vi "HardwareConfiguration.vi"() -> (3 "configured?":bool=TRUE)   [LabVIEW 2018]
uses:
  InstrControl/InstrumentSetup.vi
  globals/QC_RunInformation.vi
  InstrControl/InstrControl.lvclass
panel:
  in  "RC Configuration":u16(ring) items=["serial", "parallel"]
  in  "AC amplitude [V]":sgl=0.1
  in  "AC frequency [Hz]":i32=1000 format="%#.3p"
  in  "Matrix Configurations":bool
  in  "Defaults Multimeter":bool
  in  "Multimeter":enum32{"Keithley 2000"}(tab)
  in  "Range Value\n(0.1 - 100)":dbl=100.0 format="%#.2g"
  in  "Range":u16(ring) items=["Auto", "Manual"]
  in  "Function":u16(ring)=3 items=["AC Current", "DC Current", "AC Voltage", "DC Voltage", "2W-Resistance", "4W-Resistance", "Period", "Frequency", "Temperature", "Diode", "Continuity"]
  in  "Address KE2000":refnum<visa-resource-name>="GPIB0::19::INSTR"
  in  "Defaults LCR":bool
  in  "LCRs":T1(tab)=enum."HP4284A"
  in  "Address WK6440B":refnum<visa-resource-name>="GPIB0::6::INSTR"
  in  "Address WK6425":refnum<visa-resource-name>
  in  "Address HP4284A":refnum<visa-resource-name>="GPIB0::13::INSTR"
  in  "Consider OC":bool
  in  "Consider SC":bool
  in  "VISA address":refnum<visa-resource-name>="COM4" caption="Arduino address"
  out "Programm uploaded?":string="Make sure programme is uploaded to Arduino Uno ->"
  in  "Blank Button":bool
  in  "Supplies":T2(tab)=enum."Keithley 237"
  in  "Current Limit [µA]":sgl=100.0
  in  "Address KE2410":refnum<visa-resource-name>="GPIB0::16::INSTR"
  in  "Address KE487":refnum<visa-resource-name>
  in  "Compliance":u16(ring) items=["20µA", "2mA"]
  in  "Range:":u16(ring) items=["Autorange", "2nA", "20nA", "200nA", "2 microAmp", "20 microAmp", "200 microAmp", "2 milliAmp"]
  in  "Current Limit":u16(ring)=1 items=["OFF", "ON"]
  in  "Address KE6517":refnum<visa-resource-name>
  in  "current compliance \nlevel [mA]":dbl=0.0001 format="%.4f"
  in  "compliance/measurement\nrange (auto:0)":u16(ring)=6 items=["auto / auto", "1 nA / 1.1 V", "10 nA / 11 V", "100 nA / 110 V", "0.001 mA / 110 V", "0.01 mA / 110 V", "0.1 mA / 110 V", "1 mA / 110 V", "10 mA / 110 V", "100 mA / 110 V"]
  in  "Address KE236":refnum<visa-resource-name>
  in  "Address KE237":refnum<visa-resource-name>="GPIB0::16::INSTR"
  in  "current compliance \nlevel [uA] K237":dbl=10.0 caption="current compliance\nlevel [uA]" format="%.4f"
  in  "compliance/measurement\nrange (auto:0) K237":u16(ring) caption="compliance/measurement\nrange (auto:0)" items=["auto / auto", "1 nA / 1.1 V", "10 nA / 11 V", "100 nA / 110 V", "1 uA / 1100 V", "10 uA / *", "100 uA / *", "1 mA / *", "10 mA / *", "100 mA / *"]
  in  "Defaults Supply":bool
  in  "OK Button":bool
  # "Hardware Configuration"
  # "Multimeter Configuration"
  # "Supply Configuration"
  # "Arduino Configuration"
  # "LCR Configuration"
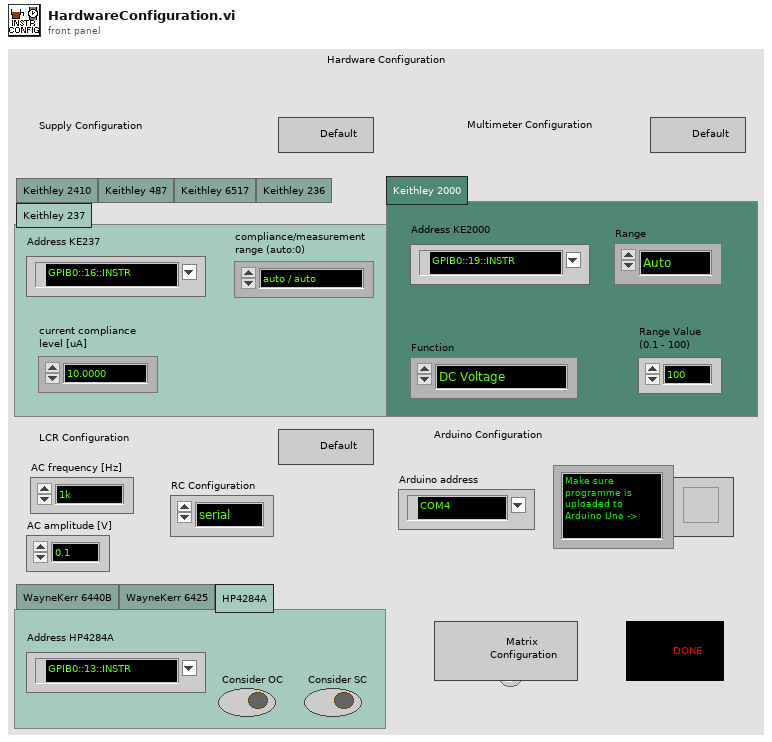
[diagram p1: front panel]
types:
  T1 = enum32{"WayneKerr 6440B", "WayneKerr 6425", "HP4284A"}
  T2 = enum32{"Keithley 2410", "Keithley 487", "Keithley 6517", "Keithley 236", "Keithley 237"}
  T3 = enum16{"CPD", "CPQ", "CPG", "CPRP", "CSD", "CSQ", "CSRS", "LPQ", "LPD", "LPG", "LPRP", "LSD", "LSQ", "LSRS", "RX", "ZTD", "ZTR", "GB", "YTD", "YTR"}
  T4 = cluster{"KE 2410":cluster{"Instrument name":string, "address":refnum<visa-resource-name>, "Instrument type":u16}, "KE 6517":cluster{"Instrument name":string, "address":refnum<visa-resource-name>, "Instrument type":u16}, "KE 487":cluster{"Instrument name":string, "address":refnum<visa-resource-name>, "Instrument type":u16}, "KE 236":cluster{"Instrument name":string, "address":refnum<visa-resource-name>, "Instrument type":u16}, "WK 6440B":cluster{"Instrument name":string, "address":refnum<visa-resource-name>, "Instrument type":u16}, "WK 6425":cluster{"Instrument name":string, "address":refnum<visa-resource-name>, "Instrument type":u16}, "Pickering Matrix":cluster{"Instrument name":string, "address":refnum<visa-resource-name>, "Instrument type":u16}, "KE 2000":cluster{"Instrument name":string, "address":refnum<visa-resource-name>, "Instrument type":u16}, "KE3706A Switching":cluster{"Instrument name":string, "address":refnum<visa-resource-name>, "Instrument type":u16}, "HP 4284A":cluster{"Instrument name":string, "address":refnum<visa-resource-name>, "Instrument type":u16}, "KE237":cluster{"Instrument name":string, "address":refnum<visa-resource-name>, "Instrument type":u16}}
  T5 = cluster{"RC Configuration":u16, "AC amplitude [V]":dbl, "AC frequency [Hz]":i32, "HP 4284A Configurations":cluster{"Consider OC":bool, "Consider SC":bool}}
  T6 = cluster{"VISA address":refnum<visa-resource-name>, "T sensor":enum16{"SHT", "DS"}, "Arduino":refnum<class "ArduinoControl.lvclass">}
  T7 = cluster{"Range":u16, "Range Value":dbl, "Function":u16, "KE2000":refnum<class "KE2000.lvclass">}
  T8 = cluster{"Current Limit":sgl, "KE2410":refnum<class "KE2410.lvclass">}
  T9 = cluster{"Compliance":u16, "Range:":u16, "KE487":refnum<class "KE487.lvclass">}
  T10 = cluster{"Current Limit":u16, "KE6517":refnum<class "KE6517.lvclass">}
  T11 = cluster{"current \ncompliance level":dbl, "compliance/\nmeasurement range (auto:0)":u16, "KE236":refnum<class "KE236.lvclass">}
  T12 = cluster{"current \ncompliance level":dbl, "compliance/\nmeasurement range (auto:0)":u16, "KE237":refnum<class "KE237.lvclass">}
  T13 = cluster{"Sensor Serial No.:":string, "Wafer:":string, "Batch:":string, "Manufacturer:":string, "Device Category:":string, "Database Serial No.:":string, "Date Initiated:":string, "Time Initiated:":string, "Test":string, "Probeplan used:":string, "End of Run Status":dbl, "End of Run comment:":string, "User:":string, "Vbias SMU":string, "LCR":string, "Test SMU":string, "Test DMM":string, "Comments":string, "Measurement results":cluster{"IV":string, "CV":string, "Cis":string, "Ris":string, "Stability":string, "PTP":string, "Striptest":string}}
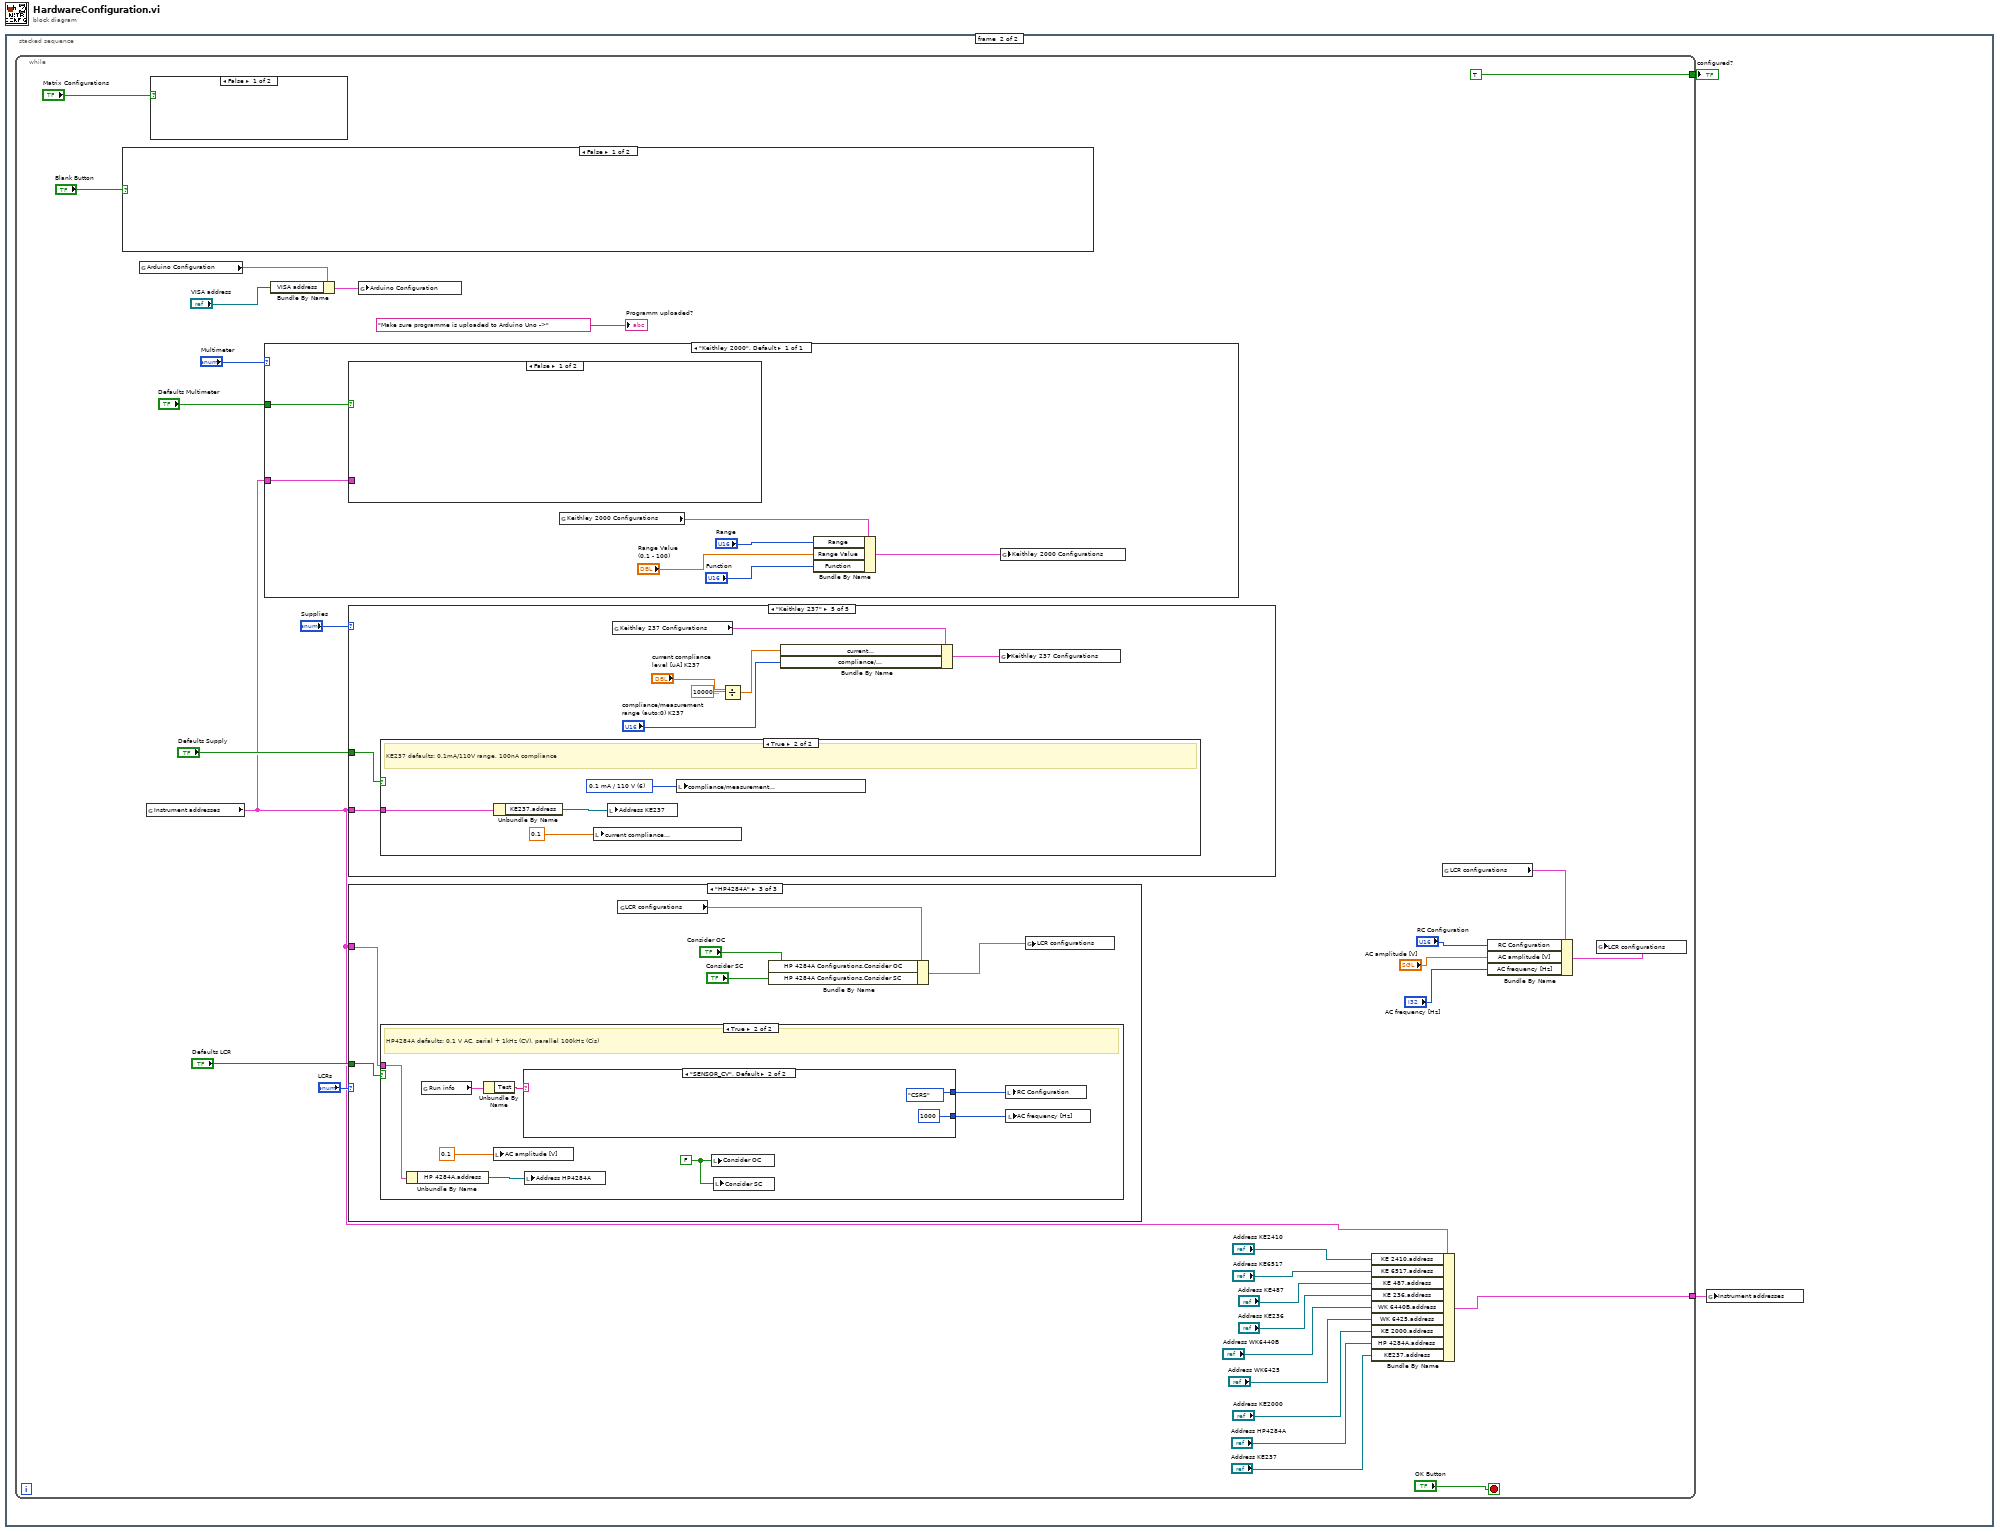
[diagram p0: block diagram]
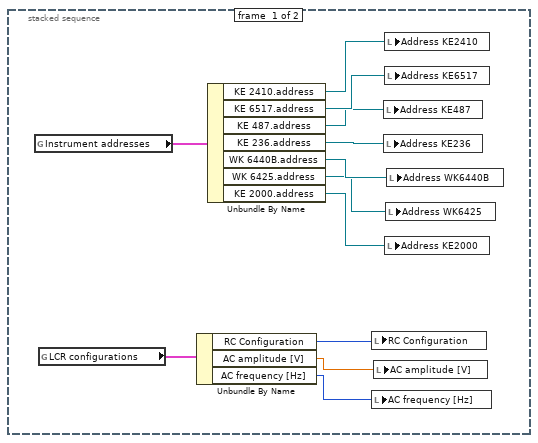
[diagram p2: hidden frame]
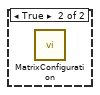
[diagram p3: hidden frame]
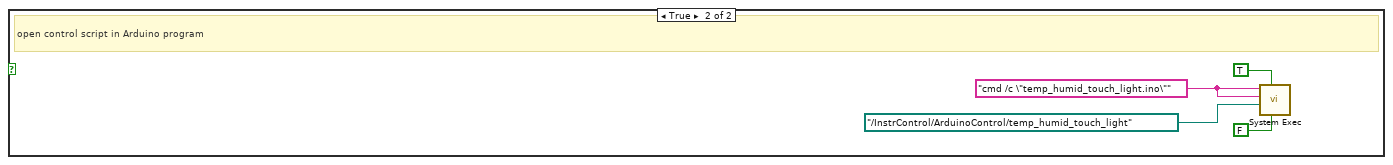
[diagram p4: hidden frame]
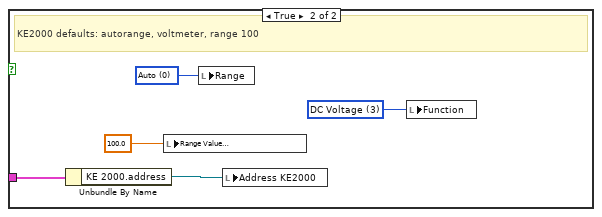
[diagram p5: hidden frame]
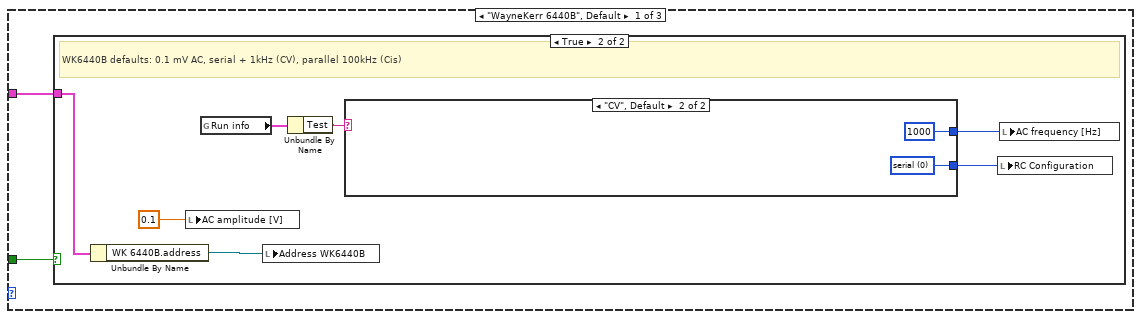
[diagram p6: hidden frame]
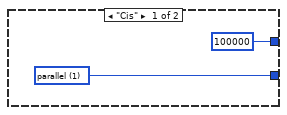
[diagram p8: hidden frame]
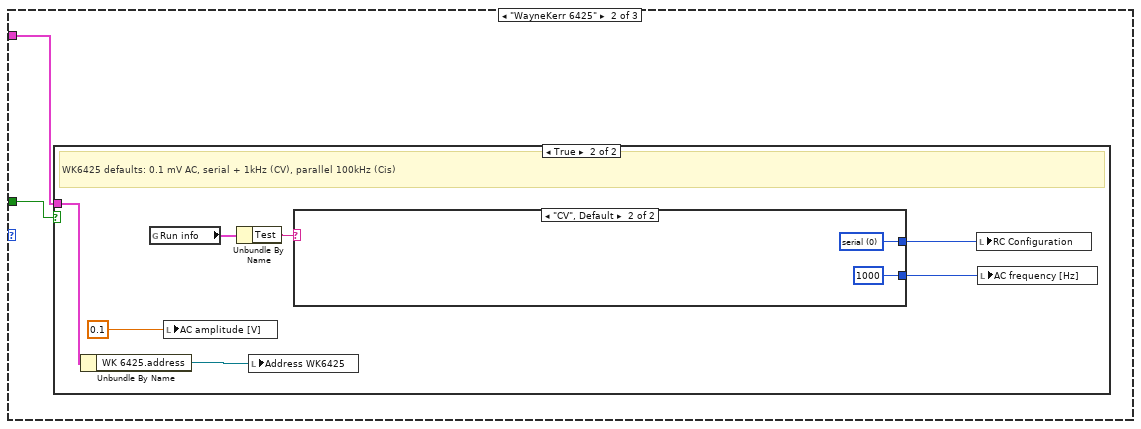
[diagram p9: hidden frame]
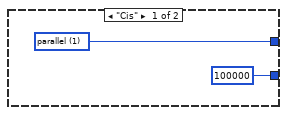
[diagram p11: hidden frame]
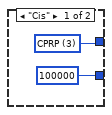
[diagram p13: hidden frame]
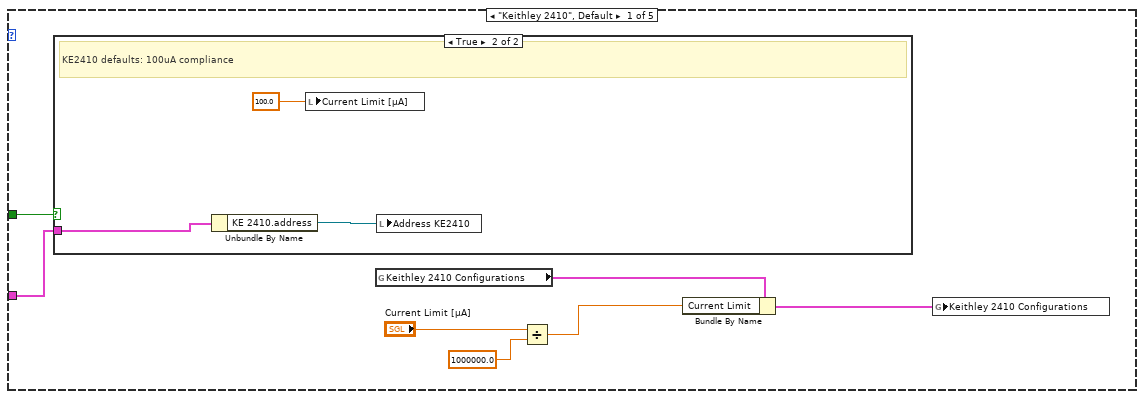
[diagram p14: hidden frame]
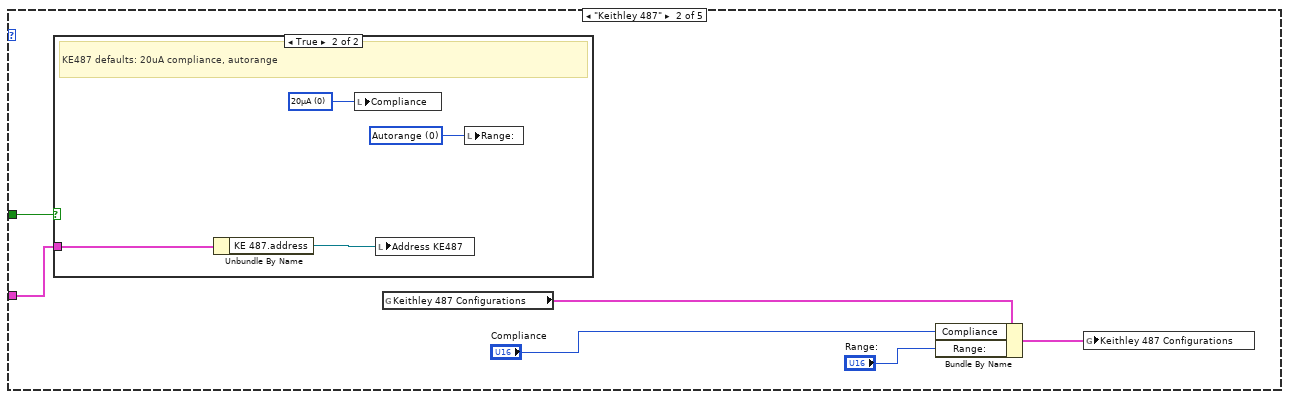
[diagram p16: hidden frame]
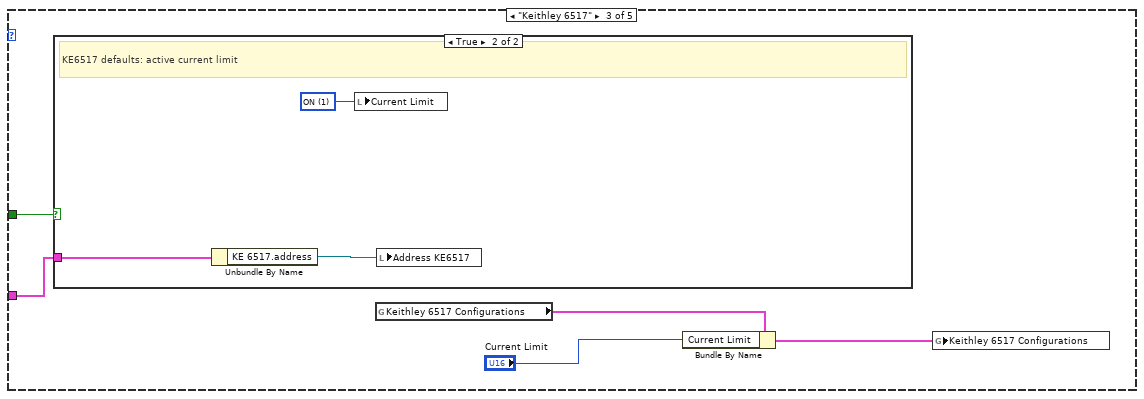
[diagram p18: hidden frame]
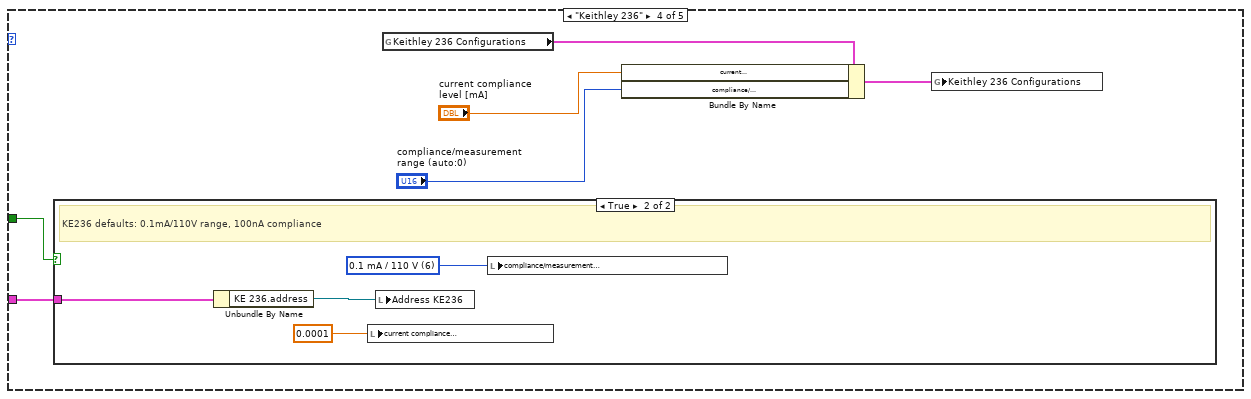
[diagram p20: hidden frame]
diagram:
  n1 = stacked-sequence {
    frame #0 {
      n2 = global read "InstrumentSetup.vi" "Instrument addresses"() -> (w12:T4)
      n3 = global read "InstrumentSetup.vi" "LCR configurations"() -> (w4:T5)
      n4 = Unbundle By Name(w4) -> ("RC Configuration"=w3:u16, "AC amplitude [V]"=w2:dbl, "AC frequency [Hz]"=w1:i32)
      n5 = Unbundle By Name(w12) -> ("KE 2410.address"=w11:refnum<visa-resource-name>, "KE 6517.address"=w10:refnum<visa-resource-name>, "KE 487.address"=w9:refnum<visa-resource-name>, "KE 236.address"=w8:refnum<visa-resource-name>, "WK 6440B.address"=w7:refnum<visa-resource-name>, "WK 6425.address"=w6:refnum<visa-resource-name>, "KE 2000.address"=w5:refnum<visa-resource-name>)
      n6 = local write "RC Configuration"(w3) -> ()
      n7 = local write "AC frequency [Hz]"(w1) -> ()
      n8 = local write "AC amplitude [V]"(w2) -> ()
      n9 = local write "Address KE487"(w9) -> ()
      n10 = local write "Address KE236"(w8) -> ()
      n11 = local write "Address KE2410"(w11) -> ()
      n12 = local write "Address KE6517"(w10) -> ()
      n13 = local write "Address KE2000"(w5) -> ()
      n14 = local write "Address WK6425"(w6) -> ()
      n15 = local write "Address WK6440B"(w7) -> ()
    }
    frame #1 {
      n16 = while {
        tunnel: [TRUE] -> w14
        tunnel: [w28] -> w13
        stop <- "OK Button" stop-if-true
        n17 = case shown="False" "Blank Button" {
          frame False {
          }
          frame True {
            w46 = "cmd /c \"temp_humid_touch_light.ino\""
            # "open control script in Arduino program"
            n18 = call <vilib>:"System Exec.vi"("run minimized? (F)"=FALSE, "wait until completion? (T)"=TRUE, "working directory"=path "../InstrControl/ArduinoControl/temp_humid_touch_light", "standard input"=w46, "command line"=w46) -> ()  [unwired: 3 in, 4 out]
          }
        }
        n19 = global read "InstrumentSetup.vi" "Arduino Configuration"() -> (w35:T6)
        n20 = global read "InstrumentSetup.vi" "Instrument addresses"() -> (w30:T4)
        n21 = case shown="False" "Matrix Configurations" {
          frame False {
          }
          frame True {
            n22 = call "MatrixConfiguration.vi"() -> ()  [unwired: 12 in]
          }
        }
        n23 = case shown="\"Keithley 2000\", Default" "Multimeter" {
          tunnel: "Defaults Multimeter" -> [w55]
          tunnel: w30 -> [w52]
          frame "Keithley 2000", Default {
            n24 = case shown="False" w55 {
              tunnel: w52 -> [_ w60]
              frame False {
              }
              frame True {
                w58 = u16 0 items=["Auto", "Manual"] ("Range")
                w59 = u16 3 items=["AC Current", "DC Current", "AC Voltage", "DC Voltage", "2W-Resistance", "4W-Resistance", "Period", "Frequency", "Temperature", "Diode", "Continuity"] ("Function")
                # "KE2000 defaults: autorange, voltmeter, range 100"
                n25 = Unbundle By Name(w60) -> ("KE 2000.address"=w56:refnum<visa-resource-name>)
                n26 = local write "Range Value\n(0.1 - 100)"(100.0 ("Range Value\n(0.1 - 100)")) -> ()
                n27 = local write "Range"(w58) -> ()
                n28 = local write "Address KE2000"(w56) -> ()
                n29 = local write "Function"(w59) -> ()
              }
            }
            n30 = global read "InstrumentSetup.vi" "Keithley 2000 Configurations"() -> (w54:T7)
            n31 = Bundle By Name(cluster=w54, "Range"="Range", "Range Value"="Range Value\n(0.1 - 100)", "Function"="Function") -> (w53:T7)
            n32 = global write "InstrumentSetup.vi" "Keithley 2000 Configurations"(w53) -> ()
          }
        }
        n33 = Bundle By Name(cluster=w35, "VISA address"="VISA address") -> (w34:T6)
        n34 = case shown="\"Keithley 237\"" "Supplies" {
          tunnel: "Defaults Supply" -> [w111 w120 w129 w138 w150]
          tunnel: w30 -> [w106 w117 w126 w135 w147]
          frame "Keithley 2410", Default {
            n35 = case shown="True" w111 {
              tunnel: w106 -> [_ w114]
              frame False {
              }
              frame True {
                # "KE2410 defaults: 100uA compliance"
                n36 = Unbundle By Name(w114) -> ("KE 2410.address"=w112:refnum<visa-resource-name>)
                n37 = local write "Current Limit [µA]"(100.0) -> ()
                n38 = local write "Address KE2410"(w112) -> ()
              }
            }
            n39 = global read "InstrumentSetup.vi" "Keithley 2410 Configurations"() -> (w110:T8)
            n40 = Divide(x="Current Limit [µA]", y=1000000.0) -> (x/y=w107:dbl)
            n41 = Bundle By Name(cluster=w110, "Current Limit"=w107) -> (w109:T8)
            n42 = global write "InstrumentSetup.vi" "Keithley 2410 Configurations"(w109) -> ()
          }
          frame "Keithley 487" {
            n43 = case shown="True" w120 {
              tunnel: w117 -> [_ w124]
              frame False {
              }
              frame True {
                w122 = u16 0 items=["Autorange", "2nA", "20nA", "200nA", "2 microAmp", "20 microAmp", "200 microAmp", "2 milliAmp"] ("Range:")
                w123 = u16 0 items=["20µA", "2mA"] ("Compliance")
                # "KE487 defaults: 20uA compliance, autorange"
                n44 = Unbundle By Name(w124) -> ("KE 487.address"=w121:refnum<visa-resource-name>)
                n45 = local write "Compliance"(w123) -> ()
                n46 = local write "Address KE487"(w121) -> ()
                n47 = local write "Range:"(w122) -> ()
              }
            }
            n48 = global read "InstrumentSetup.vi" "Keithley 487 Configurations"() -> (w119:T9)
            n49 = Bundle By Name(cluster=w119, "Compliance"="Compliance", "Range:"="Range:") -> (w118:T9)
            n50 = global write "InstrumentSetup.vi" "Keithley 487 Configurations"(w118) -> ()
          }
          frame "Keithley 6517" {
            n51 = case shown="True" w129 {
              tunnel: w126 -> [_ w132]
              frame False {
              }
              frame True {
                w131 = u16 1 items=["OFF", "ON"] ("Current Limit")
                # "KE6517 defaults: active current limit"
                n52 = Unbundle By Name(w132) -> ("KE 6517.address"=w130:refnum<visa-resource-name>)
                n53 = local write "Current Limit"(w131) -> ()
                n54 = local write "Address KE6517"(w130) -> ()
              }
            }
            n55 = global read "InstrumentSetup.vi" "Keithley 6517 Configurations"() -> (w128:T10)
            n56 = Bundle By Name(cluster=w128, "Current Limit"="Current Limit") -> (w127:T10)
            n57 = global write "InstrumentSetup.vi" "Keithley 6517 Configurations"(w127) -> ()
          }
          frame "Keithley 236" {
            n58 = case shown="True" w138 {
              tunnel: w135 -> [_ w142]
              frame False {
              }
              frame True {
                w140 = u16 6 items=["auto / auto", "1 nA / 1.1 V", "10 nA / 11 V", "100 nA / 110 V", "0.001 mA / 110 V", "0.01 mA / 110 V", "0.1 mA / 110 V", "1 mA / 110 V", "10 mA / 110 V", "100 mA / 110 V"] ("compliance/\nmeasurement range (auto:0)")
                # "KE236 defaults: 0.1mA/110V range, 100nA compliance"
                n59 = Unbundle By Name(w142) -> ("KE 236.address"=w139:refnum<visa-resource-name>)
                n60 = local write "current compliance \nlevel [mA]"(0.0001 ("current \ncompliance level")) -> ()
                n61 = local write "Address KE236"(w139) -> ()
                n62 = local write "compliance/measurement\nrange (auto:0)"(w140) -> ()
              }
            }
            n63 = global read "InstrumentSetup.vi" "Keithley 236 Configurations"() -> (w136:T11)
            n64 = Bundle By Name(cluster=w136, "current \ncompliance level"="current compliance \nlevel [mA]", "compliance/\nmeasurement range (auto:0)"="compliance/measurement\nrange (auto:0)") -> (w137:T11)
            n65 = global write "InstrumentSetup.vi" "Keithley 236 Configurations"(w137) -> ()
          }
          frame "Keithley 237" {
            n66 = case shown="True" w150 {
              tunnel: w147 -> [_ w154]
              frame False {
              }
              frame True {
                w153 = u16 6 items=["auto / auto", "1 nA / 1.1 V", "10 nA / 11 V", "100 nA / 110 V", "0.001 mA / 110 V", "0.01 mA / 110 V", "0.1 mA / 110 V", "1 mA / 110 V", "10 mA / 110 V", "100 mA / 110 V"] ("compliance/\nmeasurement range (auto:0)")
                # "KE237 defaults: 0.1mA/110V range, 100nA compliance"
                n67 = Unbundle By Name(w154) -> ("KE237.address"=w152:refnum<visa-resource-name>)
                n68 = local write "current compliance \nlevel [uA] K237"(0.1 ("current \ncompliance level")) -> ()
                n69 = local write "Address KE237"(w152) -> ()
                n70 = local write "compliance/measurement\nrange (auto:0) K237"(w153) -> ()
              }
            }
            n71 = global read "InstrumentSetup.vi" "Keithley 237 Configurations"() -> (w148:T12)
            n72 = Divide(x="current compliance \nlevel [uA] K237", y=1000000.0) -> (x/y=w144:dbl)
            n73 = Bundle By Name(cluster=w148, "current \ncompliance level"=w144, "compliance/\nmeasurement range (auto:0)"="compliance/measurement\nrange (auto:0) K237") -> (w149:T12)
            n74 = global write "InstrumentSetup.vi" "Keithley 237 Configurations"(w149) -> ()
          }
        }
        n75 = case shown="\"HP4284A\"" "LCRs" {
          tunnel: "Defaults LCR" -> [w62 w75 w90]
          tunnel: w30 -> [w61 w74 w89]
          frame "WayneKerr 6440B", Default {
            n76 = case shown="True" w62 {
              tunnel: w61 -> [_ w69]
              frame False {
              }
              frame True {
                # "WK6440B defaults: 0.1 mV AC, serial + 1kHz (CV), parallel 100kHz (Cis)"
                n77 = Unbundle By Name(w69) -> ("WK 6440B.address"=w63:refnum<visa-resource-name>)
                n78 = local write "AC amplitude [V]"(0.1) -> ()
                n79 = global read "QC_RunInformation.vi" "Run info"() -> (w65:T13)
                n80 = local write "Address WK6440B"(w63) -> ()
                n81 = Unbundle By Name(w65) -> ("Test"=w64:string)
                n82 = case shown="\"CV\", Default" w64 {
                  tunnel: [w71 w73] -> w67
                  tunnel: [100000 1000] -> w66
                  frame "Cis" {
                    w71 = u16 1 items=["serial", "parallel"] ("RC Configuration")
                  }
                  frame "CV", Default {
                    w73 = u16 0 items=["serial", "parallel"] ("RC Configuration")
                  }
                }
                n83 = local write "RC Configuration"(w67) -> ()
                n84 = local write "AC frequency [Hz]"(w66) -> ()
              }
            }
          }
          frame "WayneKerr 6425" {
            n85 = case shown="True" w75 {
              tunnel: w74 -> [_ w82]
              frame False {
              }
              frame True {
                # "WK6425 defaults: 0.1 mV AC, serial + 1kHz (CV), parallel 100kHz (Cis)"
                n86 = Unbundle By Name(w82) -> ("WK 6425.address"=w76:refnum<visa-resource-name>)
                n87 = global read "QC_RunInformation.vi" "Run info"() -> (w78:T13)
                n88 = local write "AC amplitude [V]"(0.1) -> ()
                n89 = Unbundle By Name(w78) -> ("Test"=w77:string)
                n90 = local write "Address WK6425"(w76) -> ()
                n91 = case shown="\"CV\", Default" w77 {
                  tunnel: [w84 w86] -> w80
                  tunnel: [100000 1000] -> w79
                  frame "Cis" {
                    w84 = u16 1 items=["serial", "parallel"] ("RC Configuration")
                  }
                  frame "CV", Default {
                    w86 = u16 0 items=["serial", "parallel"] ("RC Configuration")
                  }
                }
                n92 = local write "RC Configuration"(w80) -> ()
                n93 = local write "AC frequency [Hz]"(w79) -> ()
              }
            }
          }
          frame "HP4284A" {
            n94 = case shown="True" w90 {
              tunnel: w89 -> [_ w100]
              frame False {
              }
              frame True {
                w93 = FALSE
                # "HP4284A defaults: 0.1 V AC, serial + 1kHz (CV), parallel 100kHz (Cis)"
                n95 = Unbundle By Name(w100) -> ("HP 4284A.address"=w94:refnum<visa-resource-name>)
                n96 = global read "QC_RunInformation.vi" "Run info"() -> (w96:T13)
                n97 = Unbundle By Name(w96) -> ("Test"=w95:string)
                n98 = local write "AC amplitude [V]"(0.1) -> ()
                n99 = case shown="\"SENSOR_CV\", Default" w95 {
                  tunnel: [w101 T3."CSRS" ("RC Configuration HP4284A")] -> w98
                  tunnel: [100000 1000] -> w97
                  frame "Cis" {
                    w101 = u16 3 items=["CPD", "CPQ", "CPG", "CPRP", "CSD", "CSQ", "CSRS", "LPQ", "LPD", "LPG", "LPRP", "LSD", "LSQ", "LSRS", "RX", "ZTD", "ZTR", "GB", "YTD", "YTR"] ("RC Configuration HP4284A")
                  }
                  frame "SENSOR_CV", Default {
                  }
                }
                n100 = local write "Address HP4284A"(w94) -> ()
                n101 = local write "Consider OC"(w93) -> ()
                n102 = local write "Consider SC"(w93) -> ()
                n103 = local write "RC Configuration"(w98) -> ()
                n104 = local write "AC frequency [Hz]"(w97) -> ()
              }
            }
            n105 = global read "InstrumentSetup.vi" "LCR configurations"() -> (w92:T5)
            n106 = Bundle By Name(cluster=w92, "HP 4284A Configurations.Consider OC"="Consider OC", "HP 4284A Configurations.Consider SC"="Consider SC") -> (w91:T5)
            n107 = global write "InstrumentSetup.vi" "LCR configurations"(w91) -> ()
          }
        }
        n108 = global write "InstrumentSetup.vi" "Arduino Configuration"(w34) -> ()
        n109 = Bundle By Name(cluster=w30, "KE 2410.address"="Address KE2410", "KE 6517.address"="Address KE6517", "KE 487.address"="Address KE487", "KE 236.address"="Address KE236", "WK 6440B.address"="Address WK6440B", "WK 6425.address"="Address WK6425", "KE 2000.address"="Address KE2000", "HP 4284A.address"="Address HP4284A", "KE237.address"="Address KE237") -> (w28:T4)
        n110 = global read "InstrumentSetup.vi" "LCR configurations"() -> (w19:T5)
        n111 = Bundle By Name(cluster=w19, "RC Configuration"="RC Configuration", "AC amplitude [V]"="AC amplitude [V]", "AC frequency [Hz]"="AC frequency [Hz]") -> (w18:T5)
        n112 = global write "InstrumentSetup.vi" "LCR configurations"(w18) -> ()
        "Programm uploaded?" <- "Make sure programme is uploaded to Arduino Uno ->"
      }
      "configured?" <- w14
      n113 = global write "InstrumentSetup.vi" "Instrument addresses"(w13) -> ()
    }
  }
